vi "Do Read.vi"(8 "error in (no error)":errorcluster, 9 "Timeout ms":i32, 10 "Count":i32, 11 "WebSocket Client in":refnum<class "WebSocket Client.lvclass">) -> (0 "error out":errorcluster, 1 "Remaining  Timeout":i32, 2 "Data":string, 3 "WebSocket Client out":refnum<class "WebSocket Client.lvclass">)   [LabVIEW 2020, in "HTTP Server.lvlib" / "WebSocket Client.lvclass"]
uses:
  WebSocket Client.lvclass
  WebSocket Client.lvclass/WebSocket Client.ctl
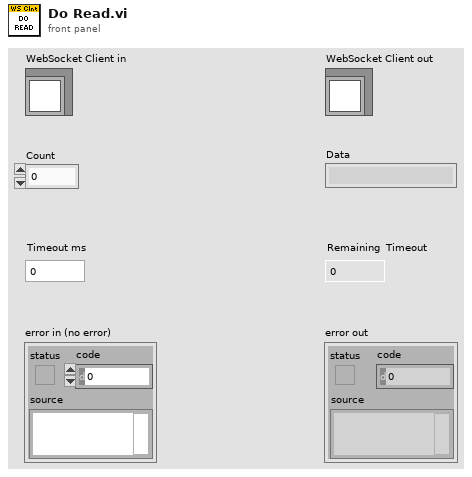
[diagram p1: front panel]
types:
  T1 = enum16{"Standard", "Buffered", "CRLF", "Immediate"}
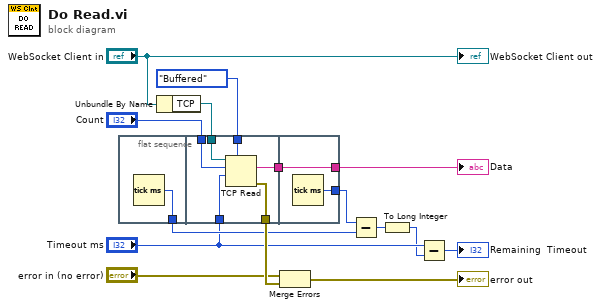
[diagram p0: block diagram]
diagram:
  n1 = flat-sequence {
    tunnel: [w16] -> w9
    tunnel: T1."Buffered" ("mode (standard)") -> [w22]
    tunnel: [w21] -> w15
    tunnel: [w20] -> w12
    tunnel: w11 -> [w19]
    tunnel: "Count" -> [w18]
    tunnel: "Timeout ms" -> [w17]
    tunnel: [w24] -> w13
    tunnel: w15 -> [w24]
    tunnel: [w23] -> w8
    frame #0 {
      n2 = Tick Count (ms)() -> (millisecond timer value=w16:u32)
    }
    frame #1 {
      n3 = TCP Read(connection ID=w19, bytes to read=w18, 7:w22, 9:w17) -> (data out=w21:string, error out=w20:errorcluster)  [unwired: 1 in, 1 out]
    }
    frame #2 {
      n4 = Tick Count (ms)() -> (millisecond timer value=w23:u32)
    }
  }
  n5 = Unbundle By Name("WebSocket Client in") -> ("TCP"=w11:refnum<k5>)
  n6 = Merge Errors("error in (no error)", w12) -> (→"error out":errorcluster)
  n7 = Subtract(x=w8, y=w9) -> (x-y=w6:u32)
  n8 = To Long Integer(number=w6) -> (32bit integer=w4:i32)
  n9 = Subtract(x="Timeout ms", y=w4) -> (x-y=→"Remaining  Timeout":i32)
  "WebSocket Client out" <- "WebSocket Client in"
  "Data" <- w13
